vi "Day 8 - Treetop Tree House.vi"() -> ()   [LabVIEW 2020, in "AoC 2022.lvlib"]
uses:
  AoC 2022.lvlib
  <vilib>/Math Plots/3D Math Plots/3D Bar/3D Bar XCtrl/3D Bar.xctl
  <vilib>/Math Plots/3D Math Plots/3D Bar/3D Bar Datatype/3D Bar Datatype.lvclass
  49fbcd14-0c67-467b-b18a-17395eff0e31.vi
  <vilib>/Math Plots/3D Math Plots/3D Bar/3D Bar Datatype/Public/Plot Helper (Matrix).vi
panel:
  in  "Puzzle Input":string="30373\n25512\n65332\n33549\n35390"
  out "3D Bar":refnum<class "3D Plot Datatype.lvclass">[](xcontrol)
  out "Puzzle Part-2 Answer":string
  out "Puzzle Answer":string
  # "Press Ctrl+M & Enter the Puzzle Input and run the VI"
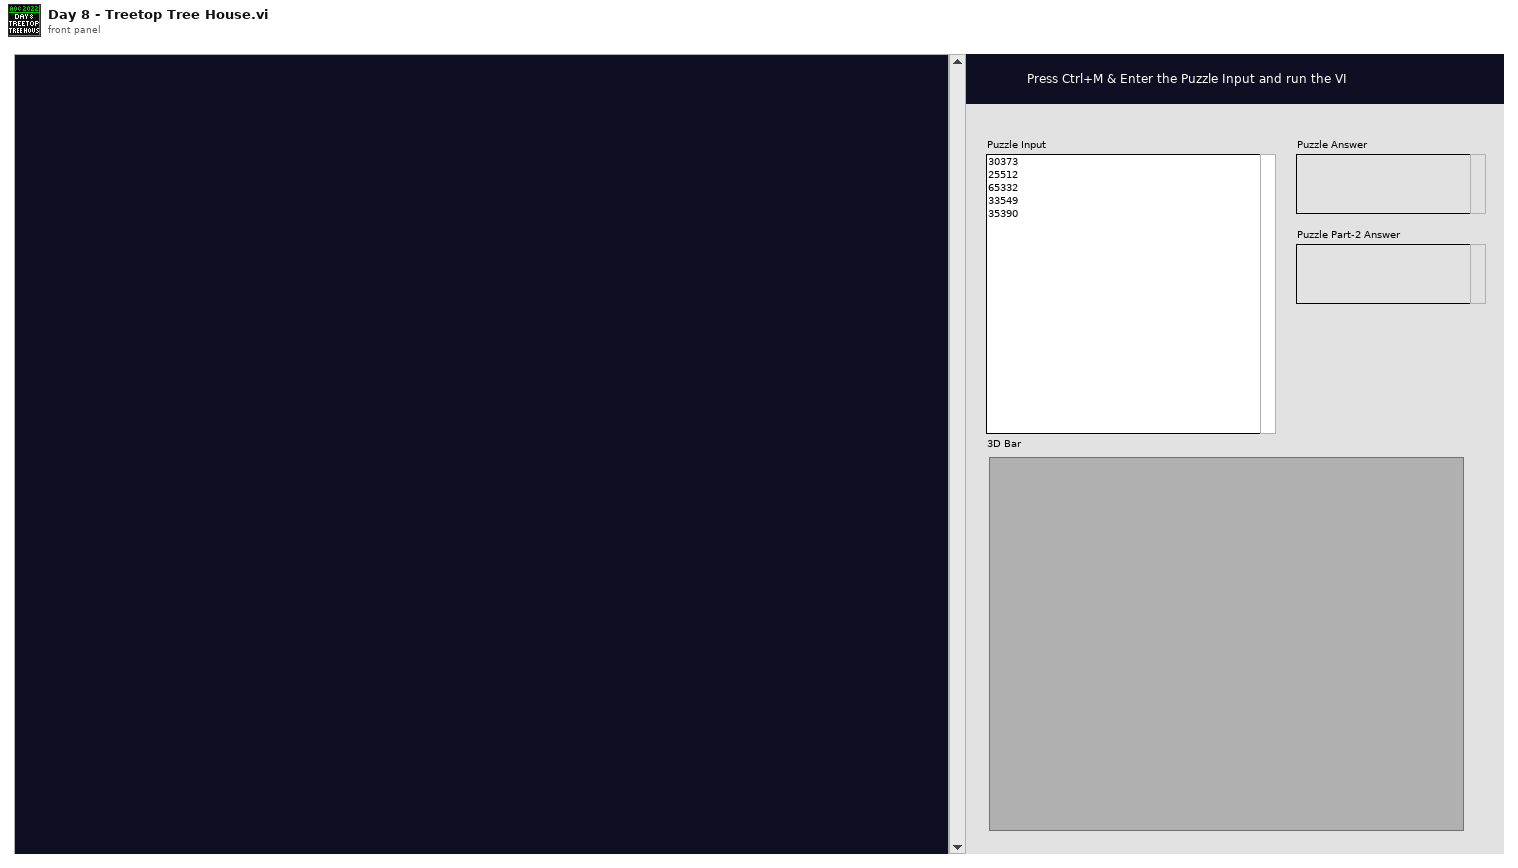
[diagram p1: front panel]
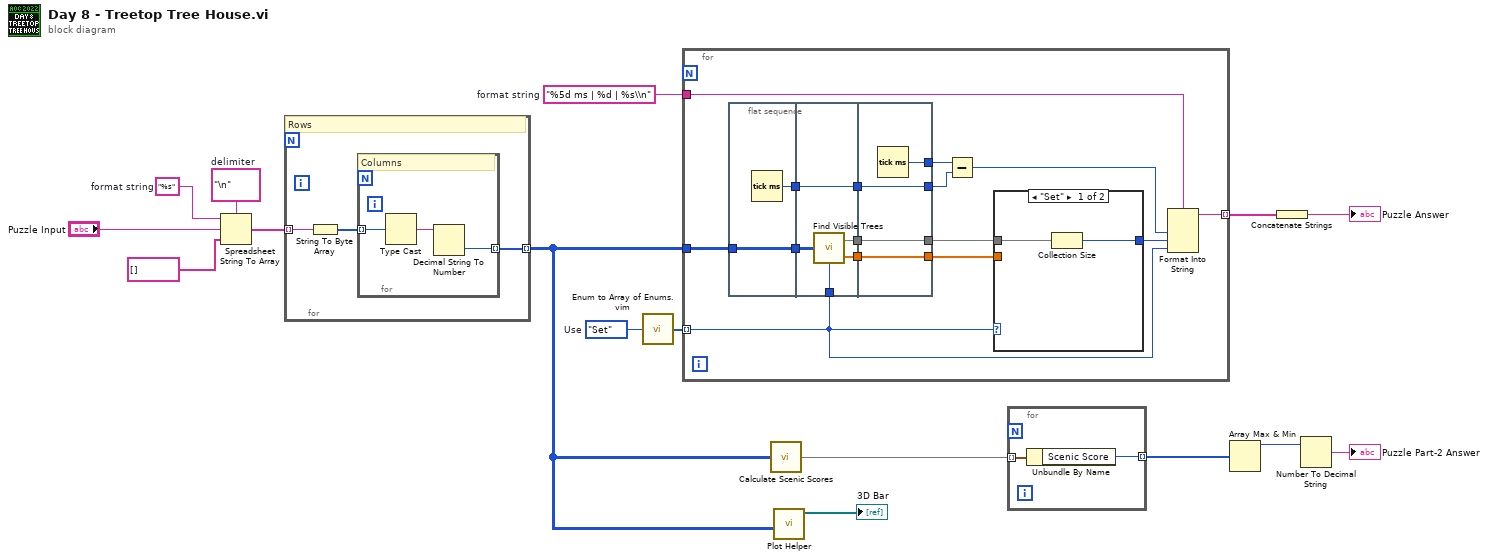
[diagram p0: block diagram]
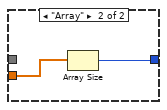
[diagram p2: hidden frame]
diagram:
  w3 = "%5d ms | %d | %s\\n"  # format string
  w7 = enum16{"Set", "Array"}."Set"  # Use
  w14 = "%s"  # format string
  w16 = "\n"  # delimiter
  n1 = Spreadsheet String To Array(delimiter (Tab)=w16, format string=w14, spreadsheet string="Puzzle Input", array type (2D Dbl)=string[] []) -> (array=w12:string[])
  n2 = for {
    tunnel: w12 -> [w19] mode=indexing
    tunnel: [w17] -> w1 mode=indexing
    # "Rows"
    n3 = String To Byte Array(string=w19) -> (unsigned byte array=w18:u8[])
    n4 = for {
      tunnel: w18 -> [w22] mode=indexing
      tunnel: [w20] -> w17 mode=indexing
      # "Columns"
      n5 = Type Cast(x=w22) -> (*(type *) &x=w21:string)  [unwired: 1 in]
      n6 = Decimal String To Number(string=w21) -> (number=w20:i32)  [unwired: 2 in, 1 out]
    }
  }
  n7 = call "Enum to Array of Enums.vim"("enum"=w7) -> ("array of enums"=w6:enum16{"Set", "Array"}[])
  n8 = for {
    tunnel: w1 -> [w37]
    tunnel: w6 -> [w32] mode=indexing
    tunnel: [w33] -> w4 mode=indexing
    tunnel: w3 -> [w23]
    n9 = flat-sequence {
      tunnel: w37 -> [w39]
      tunnel: [w39] -> w31
      tunnel: [w38] -> w27
      tunnel: w32 -> [w41]
      tunnel: w31 -> [w44]
      tunnel: [w43] -> w30
      tunnel: [w42] -> w29
      tunnel: w27 -> [w40]
      tunnel: [w40] -> w26
      tunnel: [w47] -> w35
      tunnel: [w48] -> w36
      tunnel: w30 -> [w48]
      tunnel: w29 -> [w47]
      tunnel: [w46] -> w28
      tunnel: w26 -> [w45]
      tunnel: [w45] -> w25
      frame #0 {
        n10 = Tick Count (ms)() -> (millisecond timer value=w38:u32)
      }
      frame #1 {
        n11 = call "Find Visible Trees.vi"("Tree Grid"=w44, "Use"=w41) -> ("Visible Trees (set)"=w43:set{cdb}, "Visible Trees (array)"=w42:cdb[])
      }
      frame #2 {
        n12 = Tick Count (ms)() -> (millisecond timer value=w46:u32)
      }
    }
    n13 = Subtract(x=w28, y=w25) -> (x-y=w24:u32)
    n14 = case shown="\"Set\"" w32 {
      tunnel: [w50 w51] -> w34
      tunnel: w36 -> [w49 _]
      tunnel: w35 -> [_ w52]
      frame "Set" {
        n15 = Collection Size(1:w49) -> (0:w50:i32)
      }
      frame "Array" {
        n16 = Array Size(array=w52) -> (size(s)=w51:i32)
      }
    }
    n17 = Format Into String(format string=w23, w24, w34, w32) -> (resulting string=w33:string)  [unwired: 2 in, 1 out]
  }
  n18 = call "Calculate Scenic Scores.vi"("Tree Grid"=w1) -> ("Scenic Scores"=w9:map{cdb, i32})
  n19 = call-poly <vilib>:"Plot Helper.vi"("z matrix"=w1) -> ("3D Plot lvclass Array out"=→"3D Bar":refnum<class "3D Plot Datatype.lvclass">[])  [unwired: 2 in, 8 out]
  n20 = for {
    tunnel: w9 -> [w54] mode=indexing
    tunnel: [w53] -> w10 mode=indexing
    n21 = Unbundle By Name(w54) -> ("Scenic Score"=w53:i32)
  }
  n22 = Array Max & Min(array=w10) -> (max value=w8:i32)  [unwired: 3 out]
  n23 = Concatenate Strings(w4) -> (→"Puzzle Answer":string)
  n24 = Number To Decimal String(number=w8) -> (decimal integer string=→"Puzzle Part-2 Answer":string)  [unwired: 1 in]
